vi "S2C_ExeScriptTestName.vi"(8 "Error In":errorcluster) -> (0 "Error Out":errorcluster, 2 "Canceled?":bool, 3 "Name Out":string)   [LabVIEW 2015]
doc: "Loads script data into the executable table, and resets all cells to their default colors."
panel:
  out "Init":bool
  in  "Done":bool
  in  "Name":string caption="Enter Test Name"
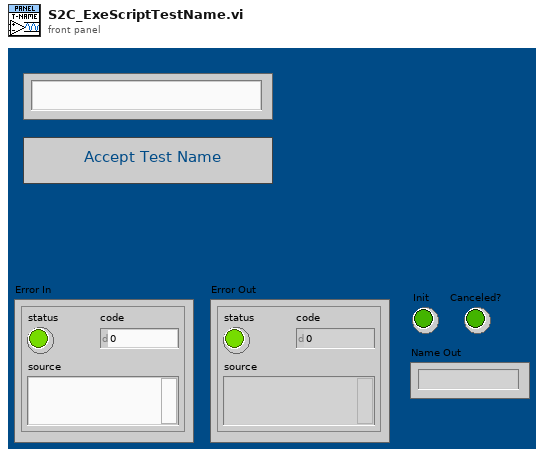
[diagram p1: front panel]
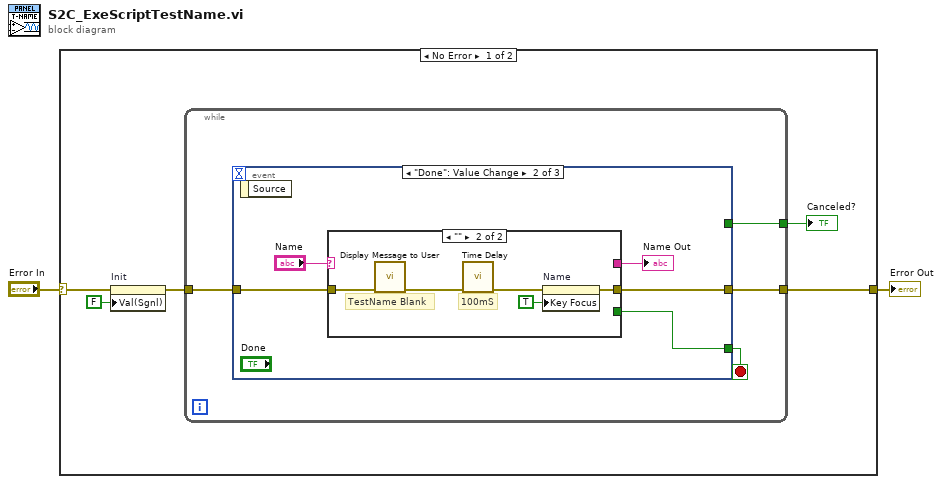
[diagram p0: block diagram]
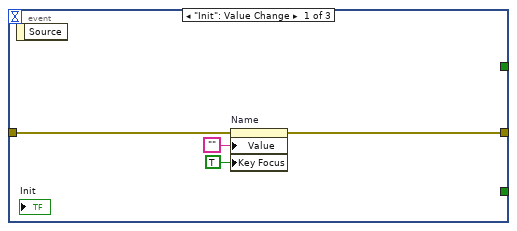
[diagram p2: hidden frame]
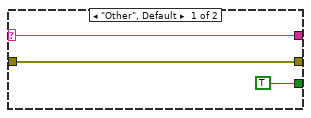
[diagram p3: hidden frame]
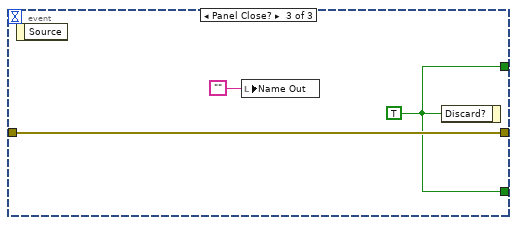
[diagram p4: hidden frame]
diagram:
  n1 = case shown="No Error" "Error In" {
    selector: "Error In" -> [w7 w32]
    tunnel: [w4 w32] -> w1
    frame No Error {
      n2 = property on="Init" class="Bool (strict)"(error in=w7, "Val(Sgnl)"=FALSE ("Value (Signaling)")) -> (error out=w5:errorcluster)  [unwired: 1 in, 1 out]
      n3 = while {
        tunnel: w5 -> [w11]
        tunnel: [w10] -> w4
        tunnel: [w8] -> w3
        stop <- w9 stop-if-true
        n4 = event shown="[1] \"Done\": Value Change" {
          selector: _ -> [_ _ _]
          dyn-events: _ -> [_ _ _]
          timeout: _ -> [_ _ _]
          tunnel: w11 -> [w13 w20 w30]
          tunnel: [w12 w18 w30] -> w10
          tunnel: [_ w17 w29] -> w9
          tunnel: [_ _ w29] -> w8
          event "Init": Value Change {
            n5 = event-data() -> ()  [unwired: 1 in, 1 out]
            n6 = property on="Name" class="Str"(error in=w13, "Value"="", "Key Focus"=TRUE) -> (error out=w12:errorcluster)  [unwired: 1 in, 1 out]
          }
          event "Done": Value Change {
            n7 = event-data() -> ()  [unwired: 1 in, 1 out]
            n8 = case shown="\"\"" "Name" {
              selector: "Name" -> [w22 _]
              tunnel: w20 -> [w23 w28]
              tunnel: [w23 w26] -> w18
              tunnel: [w22 _] -> w16
              tunnel: [TRUE ("Key Focus") _] -> w17
              frame "Other", Default {
              }
              frame "" {
                # "100mS"
                # "TestName Blank"
                n9 = call "Display Message to User"("error in (no error)"=w28) -> ("error out"=w25:errorcluster)  [unwired: 9 in, 1 out]
                n10 = call "Time Delay"("error in (no error)"=w25) -> ("error out"=w24:errorcluster)  [unwired: 10 in]
                n11 = property on="Name" class="Str"(error in=w24, "Key Focus"=TRUE) -> (error out=w26:errorcluster)  [unwired: 1 in, 1 out]
              }
            }
            "Name Out" <- w16
          }
          event Panel Close? {
            w29 = TRUE ("Discard?")
            n12 = event-data() -> ()  [unwired: 1 in, 1 out]
            n13 = local write "Name Out"("") -> ()
            n14 = event-data("Discard?"=w29) -> ()  [unwired: 1 in, 1 out]
          }
        }
      }
      "Canceled?" <- w3
    }
    frame Error {
    }
  }
  "Error Out" <- w1
